vi "Get Pending Frame Or Null.vi"(8 "error in (no error)":errorcluster, 11 "TLCamera reference":refnum<k24>) -> (0 "error out":errorcluster, 2 "Pending Frame Or Null":refnum<k24>, 3 "TLCamera reference out":refnum<k24>)   [LabVIEW 2019]
uses:
  C:/Users/jleeman/git_repos/CAxis_Machine/C-Axis LabView Controller/Library_X64/Thorlabs.TSI.TLCameraInterfaces.dll
  Library_X64/Thorlabs.TSI.TLCameraInterfaces.dll
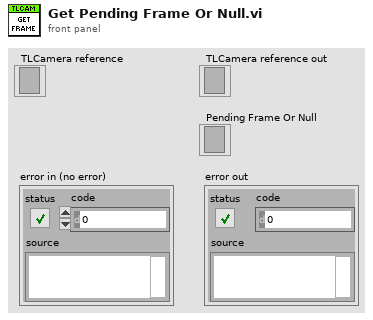
[diagram p1: front panel]
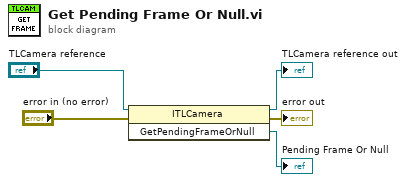
[diagram p0: block diagram]
diagram:
  n1 = invoke class="ITLCamera" method="GetPendingFrameOrNull"(reference="TLCamera reference", error in="error in (no error)") -> (reference out=→"TLCamera reference out":refnum<k24>, error out=→"error out":errorcluster, "GetPendingFrameOrNull"=→"Pending Frame Or Null":refnum<k24>)  [unwired: 1 in]
